vi "Global  pressure.vi"() -> ()   [LabVIEW 2018]
panel:
  in  "Array":dbl[](array[numeric])
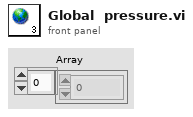
[diagram p1: front panel]
diagram:
